vi "Field to Robot Coords.vi"(9 "gyro":dbl, 10 "Joystick y":dbl, 11 "Joystick x":dbl) -> (2 "robot y":dbl, 3 "robot x":dbl)   [LabVIEW 2014]
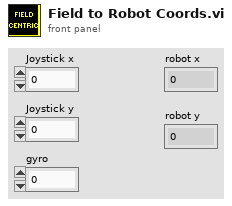
[diagram p1: front panel]
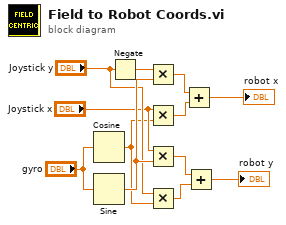
[diagram p0: block diagram]
diagram:
  n1 = Cosine(x="gyro") -> (cos(x)=w7:dbl)
  n2 = Sine(x="gyro") -> (sin(x)=w10:dbl)
  n3 = Negate(x="Joystick y") -> (-x=w6:dbl)
  n4 = Multiply(x=w6, y=w10) -> (x*y=w2:dbl)
  n5 = Multiply(x="Joystick x", y=w7) -> (x*y=w3:dbl)
  n6 = Multiply(x="Joystick x", y=w10) -> (x*y=w4:dbl)
  n7 = Multiply(x="Joystick y", y=w7) -> (x*y=w5:dbl)
  n8 = Add(x=w2, y=w3) -> (x+y=→"robot x":dbl)
  n9 = Add(x=w4, y=w5) -> (x+y=→"robot y":dbl)
